vi "ProcessCommand.vi"(5 "Ctl Refnum":refnum<vi>, 7 "Command":variant, 8 "error in (no error)":errorcluster, 9 "Data":T1=variant(string "Default"), 10 "Queue with Cluster Reference":T2, 11 "UserDefined Command class in":refnum<class "UserDefined Command class.lvclass">) -> (0 "error out":errorcluster, 2 "Queue (dup)":T2, 3 "UserDefined Command class out":refnum<class "UserDefined Command class.lvclass">)   [LabVIEW 2010, in "UserDefined Command class.lvclass"]
uses:
  UserDefined Command class.lvclass
  <userlib>/Common/Queue with Cluster/TYP_Queue with Cluster Reference.ctl
  Controls/TYP_VariantDefault.ctl
  <userlib>/Common/Queue with Cluster/Enqueue - ClusterBoth.vi
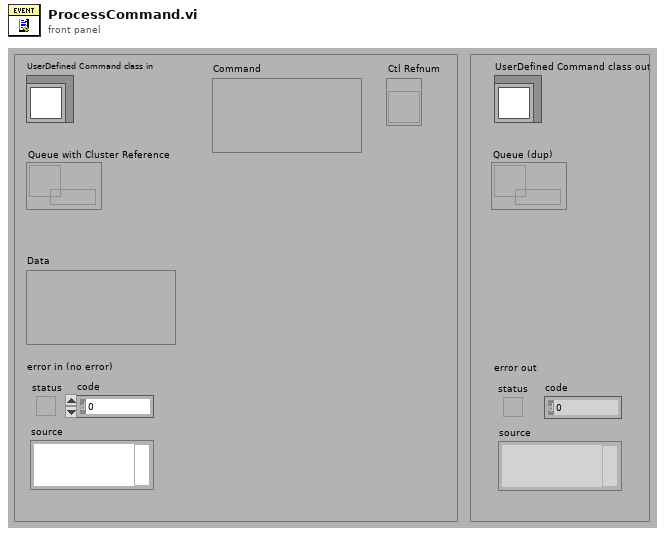
[diagram p1: front panel]
types:
  T1 = typedef "TYP_VariantDefault.ctl" = variant
  T2 = typedef "TYP_Queue with Cluster Reference.ctl" = refnum<queue>
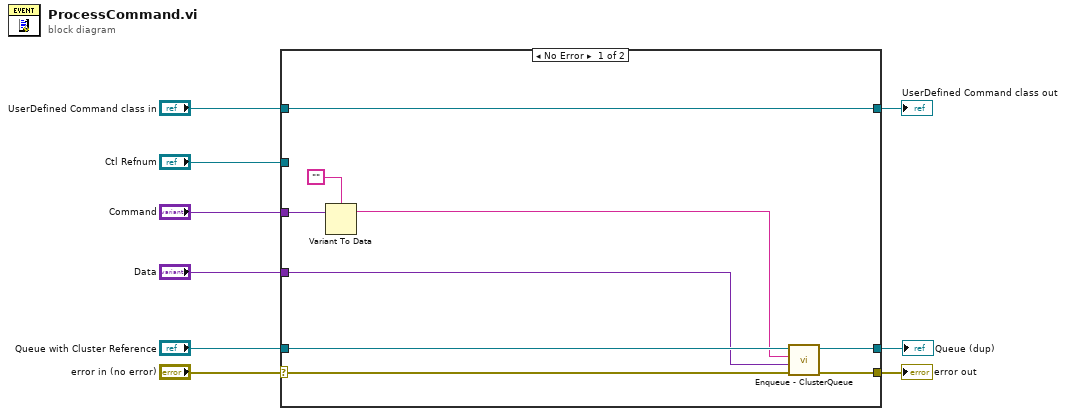
[diagram p0: block diagram]
diagram:
  n1 = case shown="No Error" "error in (no error)" {
    selector: "error in (no error)" -> [w17 w21]
    tunnel: [w16 w21] -> w8
    tunnel: [w18 w20] -> w6
    tunnel: "UserDefined Command class in" -> [w18 w20]
    tunnel: "Queue with Cluster Reference" -> [w15 w19]
    tunnel: "Command" -> [w14 _]
    tunnel: "Ctl Refnum" -> [_ _]
    tunnel: "Data" -> [w11 _]
    tunnel: [w10 w19] -> w1
    frame No Error {
      n2 = Variant To Data(Variant=w14, type="") -> (data=w12:string)  [unwired: 1 in, 1 out]
      n3 = call-poly <userlib>:"Enqueue - ClusterQueue.vi"("error in (no error)"=w17, "Data"=w11, "Command"=w12, "Queue with Cluster Reference"=w15) -> ("error out"=w16:errorcluster, "Queue Out (dup)"=w10:T2)  [unwired: 6 in]
    }
    frame Error {
    }
  }
  "error out" <- w8
  "UserDefined Command class out" <- w6
  "Queue (dup)" <- w1
